vi "brians_diode_screen.vi"(0 "Diode Charts In":T1) -> ()   [LabVIEW 2017]
uses:
  diode_charts.ctl
panel:
  out "Diode Charts Out":T1
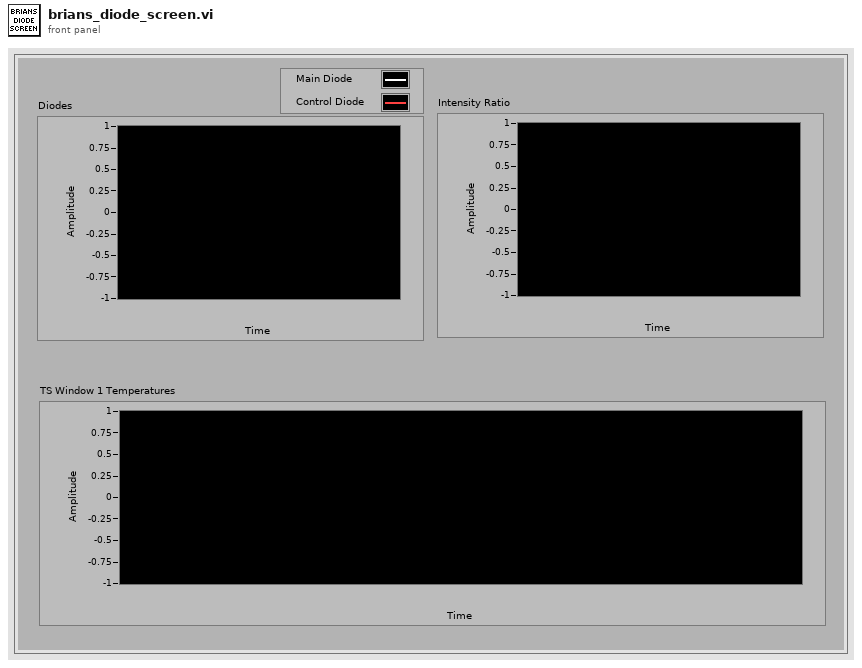
[diagram p1: front panel]
types:
  T1 = typedef "diode_charts.ctl" = cluster{"Diodes":cluster{dbl, dbl}[], "Intensity Ratio":dbl[], "TS Window 1 Temperatures":cluster{"Average":dbl, "T Sat [C]":dbl}}
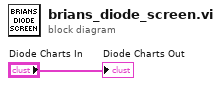
[diagram p0: block diagram]
diagram:
  "Diode Charts Out" <- "Diode Charts In"
